vi "ConvertSMUToString.vi"(11 "SMU":T1) -> (3 "Channel":string)   [LabVIEW 2013, in "Keithley-2602.lvlib"]
uses:
  Keithley-2602.lvlib
  Public/Controls/SMU.ctl
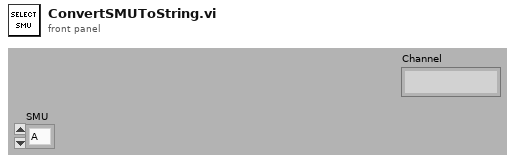
[diagram p1: front panel]
types:
  T1 = typedef "Keithley-2602.lvlib/SMU.ctl" = enum16{"A", "B"}
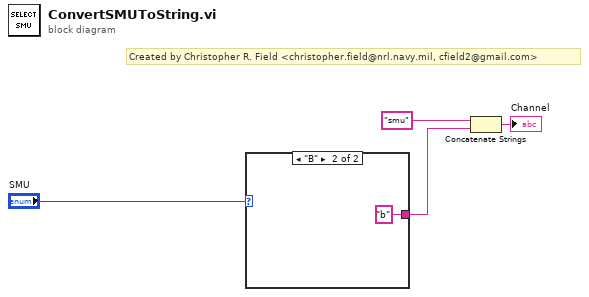
[diagram p0: block diagram]
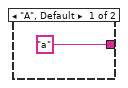
[diagram p2: hidden frame]
diagram:
  # "Created by Christopher R. Field <christopher.field@nrl.navy.mil, cfield2@gmail.com>"
  n1 = case shown="\"B\"" "SMU" {
    tunnel: ["a" "b"] -> w3
    frame "A", Default {
    }
    frame "B" {
    }
  }
  n2 = Concatenate Strings("smu", w3) -> (→"Channel":string)
